vi "Test Listen.vi"() -> ()   [LabVIEW 2014, in "Arduino SoftwareSerial Wrapper.lvlib"]
uses:
  <vilib>/Aledyne-TSXperts/Arduino Compatible Compiler for LabVIEW/addons/Arduino SoftwareSerial Wrapper/Arduino SoftwareSerial Wrapper.lvlib
panel:
  out "Is Listening? 2":bool
  out "Is Listening?":bool
  out "Error Out":errorcluster
  in  "Error In":errorcluster
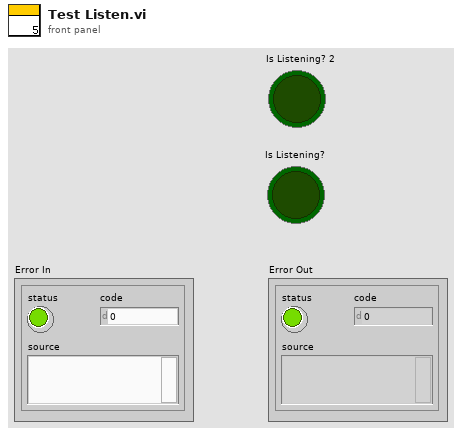
[diagram p1: front panel]
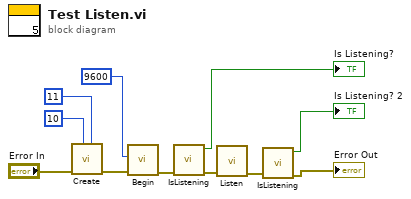
[diagram p0: block diagram]
diagram:
  n1 = call <vilib>:"Create.vi"("arduino TX pin"=u8 11, "arduino RX pin"=u8 10, "Error In"="Error In") -> ("Error Out"=w8:errorcluster)  [unwired: 8 in]
  n2 = call <vilib>:"Begin.vi"("Error In"=w8, "Baudrate"=u16 9600) -> ("Error Out"=w6:errorcluster)  [unwired: 8 in]
  n3 = call <vilib>:"IsListening.vi"("Error In"=w6) -> ("Error Out"=w5:errorcluster, "Is Listening?"=→"Is Listening?":bool)  [unwired: 9 in]
  n4 = call <vilib>:"Listen.vi"("Error In"=w5) -> ("Error Out"=w4:errorcluster)  [unwired: 10 in]
  n5 = call <vilib>:"IsListening.vi"("Error In"=w4) -> ("Error Out"=→"Error Out":errorcluster, "Is Listening?"=→"Is Listening? 2":bool)  [unwired: 9 in]
